vi "does string start with.vi"(10 "string in":string, 11 "does string start with this":string) -> (3 "Boolean":bool)   [LabVIEW 2020]
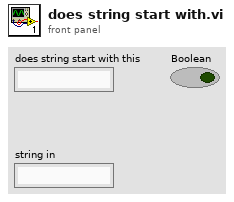
[diagram p1: front panel]
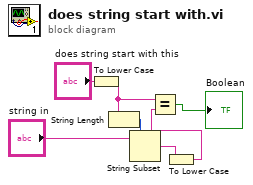
[diagram p0: block diagram]
diagram:
  n1 = To Lower Case(string="does string start with this") -> (all lower case string=w1:string)
  n2 = String Length(string=w1) -> (length=w5:i32)
  n3 = String Subset(string="string in", length (rest)=w5) -> (substring=w3:string)  [unwired: 1 in]
  n4 = To Lower Case(string=w3) -> (all lower case string=w6:string)
  n5 = Equal?(x=w1, y=w6) -> (x = y?=→"Boolean":bool)
